vi "INI Read write Dbl2dArry.vi"(5 "key":string, 7 "section":string, 8 "error in":errorcluster, 9 "Default":string="0,0,0:0,0,0", 10 "dbl array in":dbl[][](array[numeric]) format="%.2f", 11 "Read|Write":T1) -> (0 "error out":errorcluster, 2 "dbl array out":dbl[][](array[numeric]) format="%.2f")   [LabVIEW 2013]
doc: "This .vi reads/writes a double to the config file. During Write, \"dbl in\" is passed to \"dbl out\""
uses:
  Read write mode.ctl
  <vilib>/Utility/config.llb/Read Key (String).vi
  <vilib>/Utility/config.llb/Write Key (String).vi
  <vilib>/Utility/config.llb/NI_LVConfig.lvlib
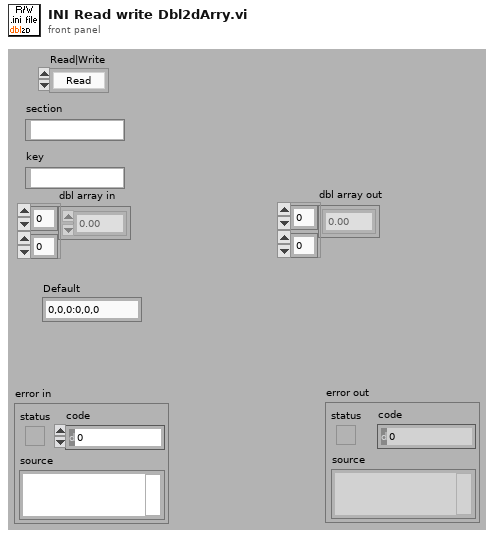
[diagram p1: front panel]
types:
  T1 = typedef "Read write mode.ctl" = enum16{"Read", "Write"}
  T2 = typedef "Semaphore RefNum" = refnum<k1>
  T3 = typedef "NI_LVConfig.lvlib/Config Data RefNum.ctl" = refnum<k1>
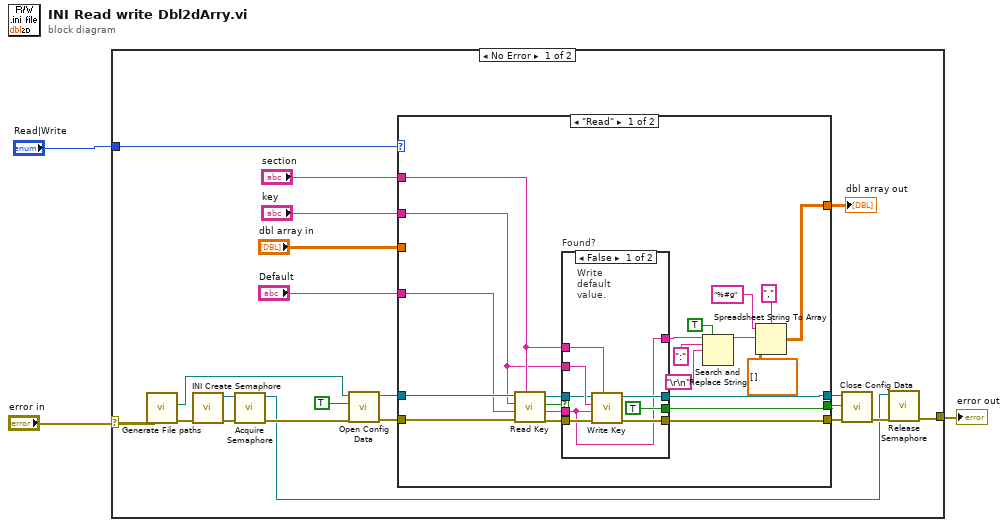
[diagram p0: block diagram]
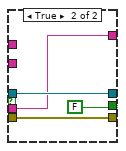
[diagram p2: hidden frame]
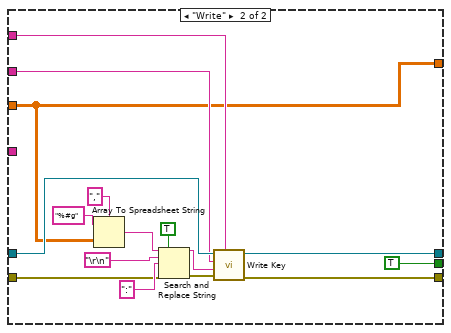
[diagram p3: hidden frame]
diagram:
  n1 = case shown="No Error" "error in" {
    selector: "error in" -> [_ w73]
    tunnel: "Read|Write" -> [w23 _]
    tunnel: [w6 w73] -> w1
    frame No Error {
      n2 = call "Generate File paths.vi"() -> ("error out"=w5:errorcluster, ".ini path"=w4:path)  [unwired: 1 in, 9 out]
      n3 = call "INI Create Semaphore.vi"("error in"=w5) -> ("error out"=w11:errorcluster, "semaphore"=w10:T2)  [unwired: 1 in, 4 out]
      n4 = call <vilib>:"Acquire Semaphore.vi"("error in (no error)"=w11, "semaphore"=w10) -> ("error out"=w9:errorcluster, "semaphore out"=w7:T2)  [unwired: 1 in, 3 out]
      n5 = call <vilib>:"Open Config Data.vi"("error in (no error)"=w9, "create file if necessary (T)"=TRUE ("create file if necessary? (T)"), "configuration file path"=w4) -> ("error out"=w18:errorcluster, "refnum"=w21:T3)  [unwired: 6 in, 1 out]
      n6 = case shown="\"Read\"" w23 {
        tunnel: [w40 w71] -> w20
        tunnel: w21 -> [w44 w72]
        tunnel: [w36 w70] -> w19
        tunnel: w18 -> [w43 w61]
        tunnel: "section" -> [w39 w69]
        tunnel: "key" -> [w38 w68]
        tunnel: [w25 w59] -> w15
        tunnel: "dbl array in" -> [_ w59]
        tunnel: [w34 TRUE ("write configuration file? (T)")] -> w13
        tunnel: "Default" -> [w42 _]
        frame "Read" {
          n7 = call-poly <vilib>:"Read Key.vi"("section"=w39, "error in (no error)"=w43, "default value"=w42, "key"=w38, "refnum"=w44) -> ("error out"=w41:errorcluster, "value"=w33:string, "found?"=w37:bool, "refnum out"=w35:T3)  [unwired: 1 in, 2 out]
          n8 = case "Found?" shown="False" w37 {
            tunnel: w41 -> [w52 w56]
            tunnel: [w51 w56] -> w40
            tunnel: w35 -> [w47 w55]
            tunnel: [w50 w55] -> w36
            tunnel: w39 -> [w49 _]
            tunnel: w38 -> [w48 _]
            tunnel: [TRUE ("write configuration file? (T)") FALSE ("write configuration file? (T)")] -> w34
            tunnel: w33 -> [w45 w53]
            tunnel: [w45 w53] -> w26
            frame False {
              # "Write\ndefault\nvalue."
              n9 = call-poly <vilib>:"Write Key.vi"("section"=w49, "error in (no error)"=w52, "value"=w45, "key"=w48, "refnum"=w47) -> ("error out"=w51:errorcluster, "refnum out"=w50:T3)  [unwired: 1 in, 4 out]
            }
            frame True {
            }
          }
          n10 = Search and Replace String(replace all?=TRUE ("replace all? (F)"), input string=w26, search string=":" ("replace string (\"\")"), replace string="\r\n") -> (result string=w31:string)  [unwired: 4 in, 3 out]
          n11 = Spreadsheet String To Array(delimiter (Tab)=",", format string="%#g", spreadsheet string=w31, array type (2D Dbl)=dbl[][] []) -> (array=w25:dbl[][])
        }
        frame "Write" {
          n12 = Array To Spreadsheet String(delimiter (Tab)=",", array=w59, 3:"%#g" ("format string")) -> (spreadsheet string=w63:string)
          n13 = Search and Replace String(replace all?=TRUE ("replace all? (F)"), input string=w63, search string="\r\n", replace string=":" ("replace string (\"\")"), error in=w61) -> (result string=w57:string, error out=w60:errorcluster)  [unwired: 3 in, 2 out]
          n14 = call-poly <vilib>:"Write Key.vi"("section"=w69, "error in (no error)"=w60, "value"=w57, "key"=w68, "refnum"=w72) -> ("error out"=w71:errorcluster, "refnum out"=w70:T3)  [unwired: 1 in, 4 out]
        }
      }
      "dbl array out" <- w15
      n15 = call <vilib>:"Close Config Data.vi"("error in (no error)"=w20, "write file if changed (T)"=w13, "refnum"=w19) -> ("error out"=w8:errorcluster)  [unwired: 8 out]
      n16 = call <vilib>:"Release Semaphore.vi"("error in (no error)"=w8, "semaphore"=w7) -> ("error out"=w6:errorcluster)  [unwired: 5 out]
    }
    frame Error {
    }
  }
  "error out" <- w1
